vi "scaling matrix_poupup.vi"() -> (0 "changed":bool, 1 "scale\nfactor":dbl, 2 "scale matrix 2":dbl[][](array[numeric])=[[1000.0, -1000.0, 200000.0, 1.0, 1.0, 1.0], [2000.0, -500.0, 1000000.0, 0.0, 0.0, 0.0], [5000.0, -1000.0, 1000000.0, 0.0, 0.0, 0.0], [10000.0, -2000.0, 1000000.0, 0.0, 0.0, 0.0], [20000.0, -5000.0, 1000000.0, 0.0, 0.0, 0.0], [500.0, -1000.0, 0.0, 0.0, 0.0, 0.0], [500.0, -40000.0, 0.0, 0.0, 0.0, 0.0], [500.0, -45000.0, 0.0, 0.0, 0.0, 0.0], [500.0, -50000.0, 0.0, 0.0, 0.0, 0.0], [500.0, -1000.0, 0.0, 0.0, 0.0, 0.0], [2000.0, -2000.0, 0.0, 0.0, 0.0, 0.0], [2000.0, -2000.0, 0.0, 0.0, 0.0, 0.0], [4000.0, -4000.0, 0.0, 0.0, 0.0, 0.0], [4000.0, -4000.0, 0.0, 0.0, 0.0, 0.0]] format="%#_6e", 3 "Scale 2":u16(ring) items=["no scaling", "universal scale", "1st row", "matrix", "frequency (matrix)", "freq. 1st col. (real 1, im 1, re 2, im 2, ....)"], 4 "x-scale":dbl=1.0)   [LabVIEW 2019]
panel:
  in  "universal x-scale":dbl=1.0
  in  "Cancel button":bool
  in  "OK Button":bool
  in  "universal y-scale":dbl
  in  "col index":i32
  in  "row index":i32
  in  "Scale":u16(ring) items=["no scaling", "universal scale", "1st row", "matrix", "frequency (matrix)", "freq. 1st col. (real 1, im 1, re 2, im 2, ....)"]
  in  "scale matrix":dbl[][](array[numeric])=[[1000.0, -1000.0, 200000.0, 1.0, 1.0, 1.0], [2000.0, -500.0, 1000000.0, 0.0, 0.0, 0.0], [5000.0, -1000.0, 1000000.0, 0.0, 0.0, 0.0], [10000.0, -2000.0, 1000000.0, 0.0, 0.0, 0.0], [20000.0, -5000.0, 1000000.0, 0.0, 0.0, 0.0], [500.0, -1000.0, 0.0, 0.0, 0.0, 0.0], [500.0, -40000.0, 0.0, 0.0, 0.0, 0.0], [500.0, -45000.0, 0.0, 0.0, 0.0, 0.0], [500.0, -50000.0, 0.0, 0.0, 0.0, 0.0], [500.0, -1000.0, 0.0, 0.0, 0.0, 0.0], [2000.0, -2000.0, 0.0, 0.0, 0.0, 0.0], [2000.0, -2000.0, 0.0, 0.0, 0.0, 0.0], [4000.0, -4000.0, 0.0, 0.0, 0.0, 0.0], [4000.0, -4000.0, 0.0, 0.0, 0.0, 0.0]] format="%#_6e"
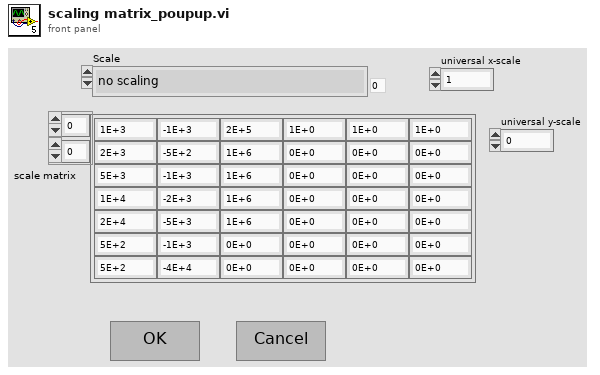
[diagram p1: front panel]
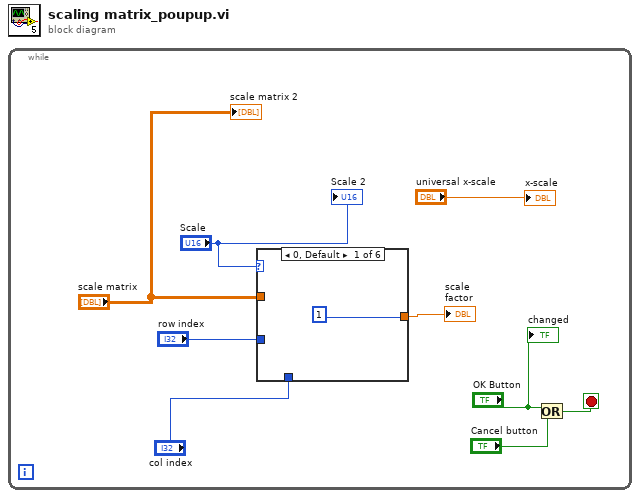
[diagram p0: block diagram]
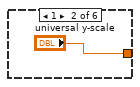
[diagram p2: hidden frame]
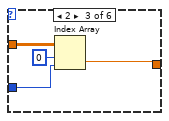
[diagram p3: hidden frame]
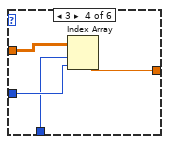
[diagram p4: hidden frame]
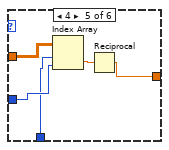
[diagram p5: hidden frame]
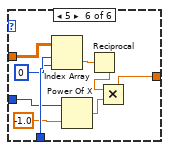
[diagram p6: hidden frame]
diagram:
  n1 = while {
    stop <- w9 stop-if-true
    n2 = case shown="0, Default" "Scale" {
      tunnel: [1 "universal y-scale" w12 w16 w20 w25] -> w2
      tunnel: "row index" -> [_ _ w13 w19 w23 w28]
      tunnel: "scale matrix" -> [_ _ w15 w17 w24 w33]
      tunnel: "col index" -> [_ _ _ w18 w22 w32]
      frame 0, Default {
      }
      frame 1 {
      }
      frame 2 {
        n3 = Index Array(array=w15, index (row)=0, index (col)=w13) -> (element=w12:dbl)
      }
      frame 3 {
        n4 = Index Array(array=w17, index (row)=w18, index (col)=w19) -> (element=w16:dbl)
      }
      frame 4 {
        n5 = Index Array(array=w24, index (row)=w22, index (col)=w23) -> (element=w21:dbl)
        n6 = Reciprocal(x=w21) -> (1/x=w20:dbl)
      }
      frame 5 {
        n7 = Index Array(array=w33, index (row)=w32, index (col)=0 ("disabled index (col)")) -> (element=w31:dbl)
        n8 = Power Of X(1:-1.0 ("x"), 2:w28) -> (0:w27:dbl)
        n9 = Reciprocal(x=w31) -> (1/x=w26:dbl)
        n10 = Multiply(x=w26, y=w27) -> (x*y=w25:dbl)
      }
    }
    "scale\nfactor" <- w2
    n11 = Or(x="OK Button", y="Cancel button") -> (x .or. y?=w9:bool)
    "scale matrix 2" <- "scale matrix"
    "changed" <- "OK Button"
    "Scale 2" <- "Scale"
    "x-scale" <- "universal x-scale"
  }
